vi "get1D.vi"(8 "error in (no error)":errorcluster caption="错误输入（无错误）", 10 "±í†Î”µ“þ":T1, 11 "HttpClient 输入":refnum<class "Http.lvclass"> caption="DNL_LabVIEW Object in") -> (0 "error out":errorcluster caption="错误输出", 2 "数组":string[](array[string]), 3 "HttpClient 输出":refnum<class "Http.lvclass"> caption="DNL_LabVIEW Object out")   [LabVIEW 2012, in "Http.lvclass"]
uses:
  Http.lvclass
  HttpData.ctl
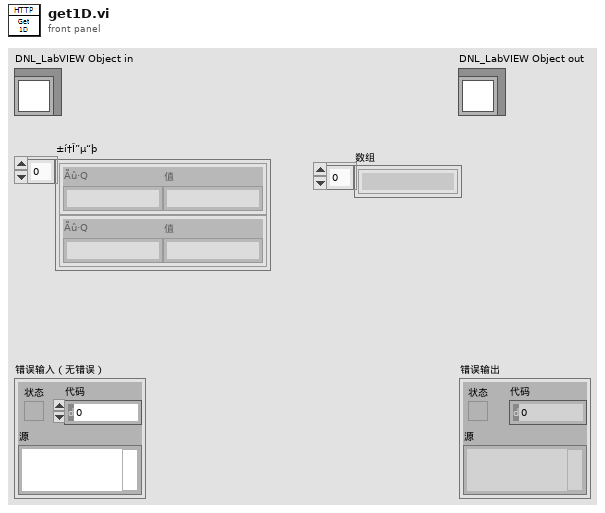
[diagram p1: front panel]
types:
  T1 = typedef "Http.lvclass/HttpData.ctl" = cluster{"Ãû·Q":string, "值":string}[]
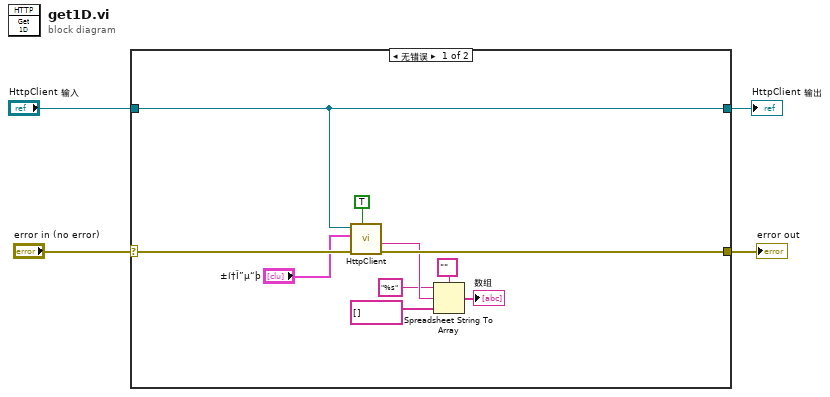
[diagram p0: block diagram]
diagram:
  n1 = case shown="无错误" "error in (no error)" {
    selector: "error in (no error)" -> [w14 w16]
    tunnel: [w13 w16] -> w3
    tunnel: [w12 w15] -> w1
    tunnel: "HttpClient 输入" -> [w12 w15]
    frame No Error {
      n2 = call-dynamic "HttpClient.vi"("™z²é î‘B?"=TRUE, "error in (no error)"=w14, "±í†Î”µ“þ"="±í†Î”µ“þ", "HttpClient 输入"=w12) -> ("error out"=w13:errorcluster, "”µ“þ"=w9:string)  [unwired: 2 in, 4 out]
      n3 = Spreadsheet String To Array(delimiter (Tab)="" ("分隔符(Tab)"), format string="%s" ("格式字符串"), spreadsheet string=w9, array type (2D Dbl)=string[] []) -> (array=→"数组":string[])
    }
    frame Error {
    }
  }
  "error out" <- w3
  "HttpClient 输出" <- w1
